vi "Reactor.vi"() -> ()   [LabVIEW 2017, in "HMILibrary.lvlib"]
uses:
  HMILibrary.lvlib
  <vilib>/Platform/TimedLoop/XDataNode/timing_clust.ctl
  <vilib>/Platform/TimedLoop/XDataNode/nitl_modes.ctl
  <vilib>/Platform/TimedLoop/XDataNode/wakeup.ctl
  <vilib>/Utility/file.llb/Write Delimited Spreadsheet (string).vi
  <vilib>/Utility/file.llb/Write Delimited Spreadsheet (DBL).vi
  <vilib>/platform/TimedLoop/XDataNode/XDataNode.xnode
  <vilib>/Platform/TimedLoop/XDataNode/XDNodeRunTimeDep.lvlib
panel:
  out "Hot Leg Temp":dbl
  out "color2":u32(colorbox)
  in  "Reactor\nPower":dbl(slide) scale=10.0..10000.0
  out "Heater Outlet Temp":dbl caption="C"
  out "Primary HX Outlet Temp":dbl
  out "Cold Leg Temp":dbl
  in  "stop":bool
  out "Warnings":string
  out "color1":u32(colorbox)
  in  "Tthreshold1":dbl=0.588
  in  "Tthreshold2":dbl=0.5934
  in  "Tthreshold3":dbl=1.6494
  in  "Tthreshold4":dbl=0.4812
  in  "dTthreshold1":dbl=2.361
  in  "dTthreshold2":dbl=2.6736
  in  "dTthreshold3":dbl=2.8362
  in  "dTthreshold4":dbl=2.1702
  in  "Tsamplethreshold":dbl=3.0
  in  "dTsamplethreshold":dbl=10.0
  out "color3":u32(colorbox)
  out "color4":u32(colorbox)
  out "Sensor 1":cluster{"placeholder1":dbl, dbl}(graph)
  out "Sensor 2":cluster{"placeholder1":dbl, dbl}(graph)
  out "Sensor 3":cluster{"placeholder1":dbl, dbl}(graph)
  out "Sensor 4":cluster{"placeholder1":dbl, dbl}(graph)
  in  "Hold Model Inputs Constant":bool
  in  "Clear Warnings":bool
  in  "Weight of measured values in filter":dbl=0.01
  # "Reactor and Primary Loop"
  # "Primary Heat\nExchanger"
  # "Reactor"
  # "Pump"
  # "Temperatures in degrees C"
  # "Fault Detection"
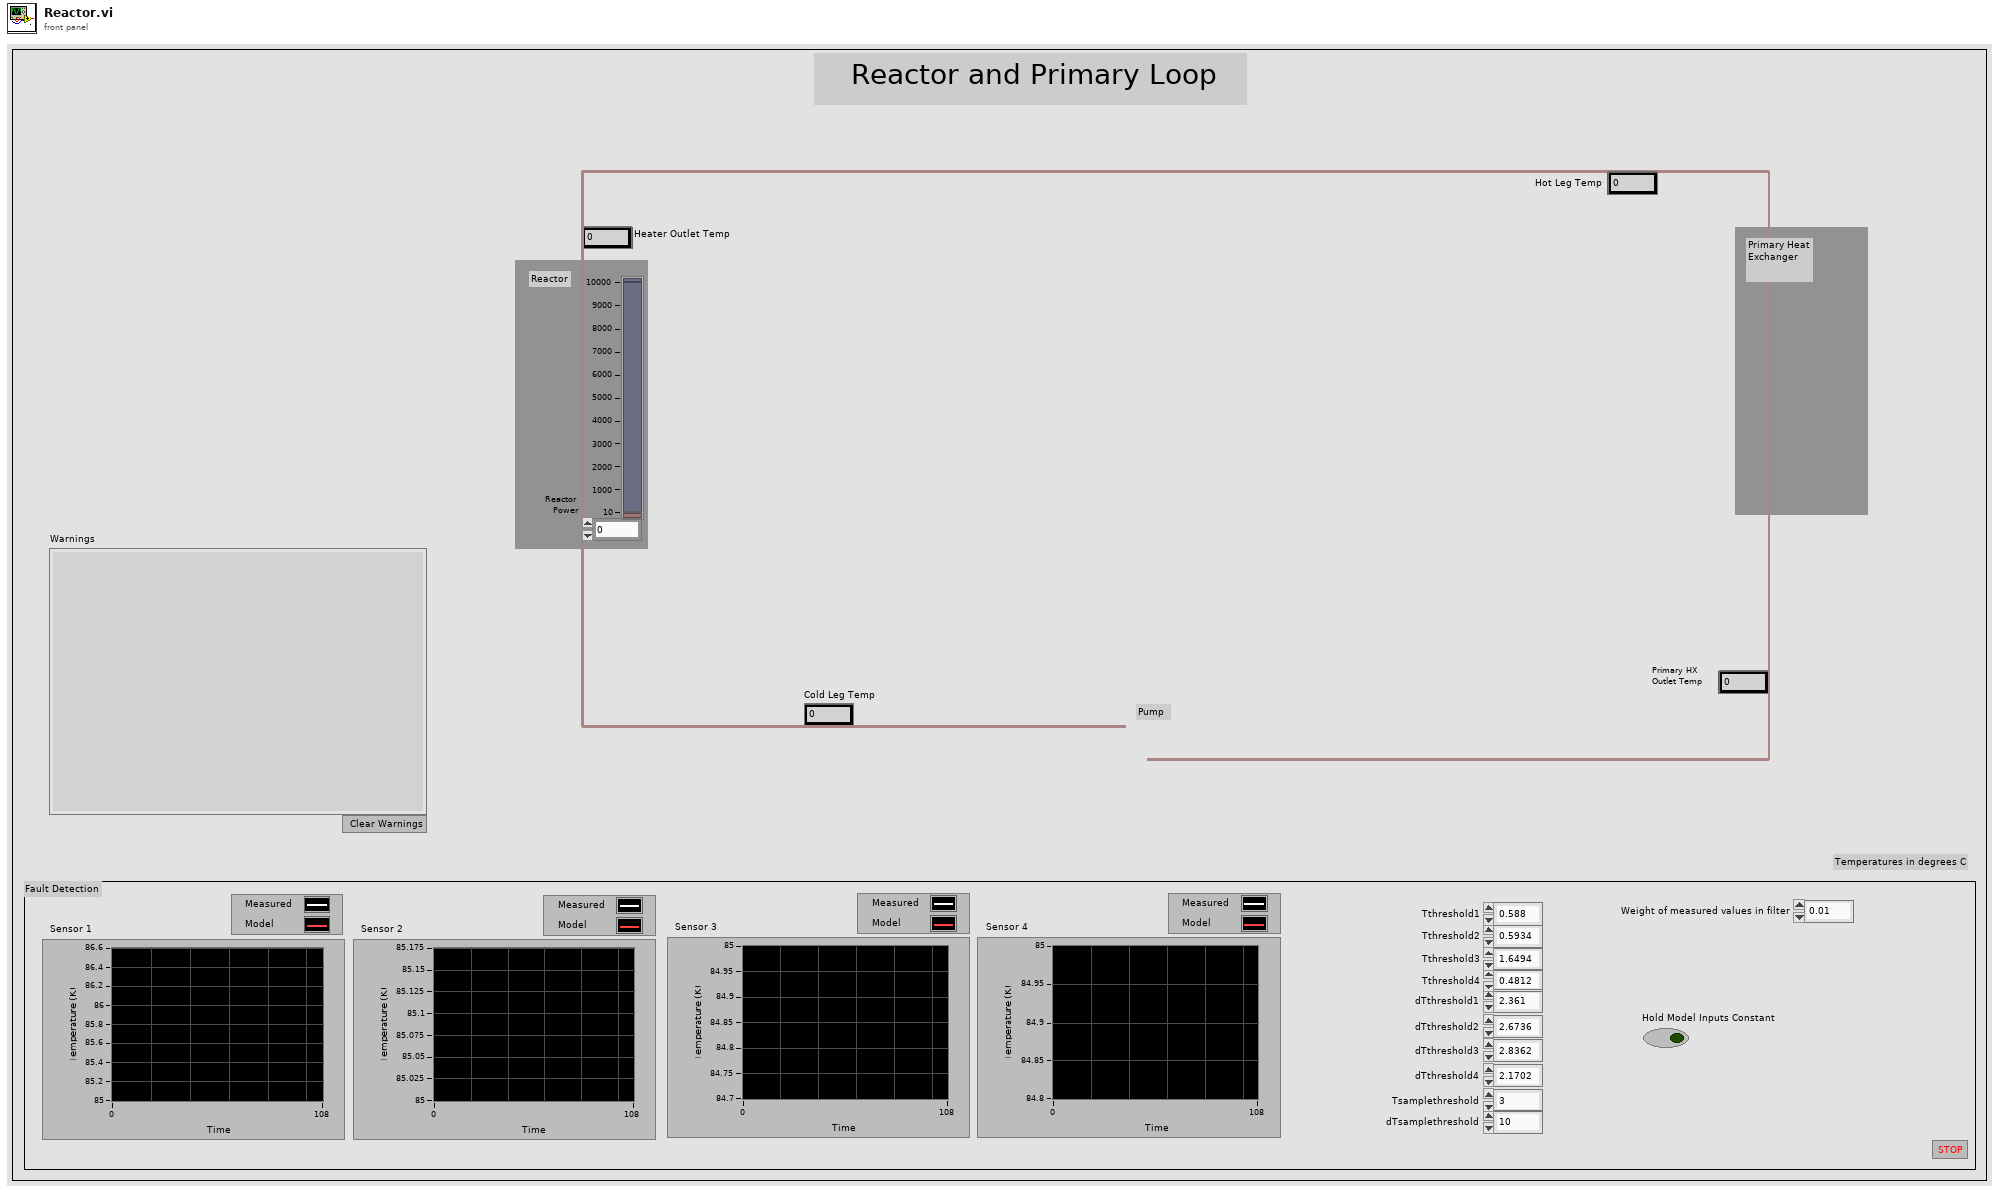
[diagram p1: front panel]
types:
  T1 = typedef "XDNodeRunTimeDep.lvlib/timing_clust.ctl" = cluster{"Expected End [f-1]":u64, "Actual End [f-1]":u64, "Finished Late? [f-1]":bool, "Expected End [i-1]":u64, "Actual End [i-1]":u64, "Finished Late? [i-1]":bool, "Expected Start [i]":u64, "Actual Start [i]":u64, "Expected Start [f]":u64, "Actual Start [f]":u64, "Source Name":string, "Structure Name":string, "Period":i64, "Deadline":i64, "Offset":i64, "Start":i64, "Priority":i32, "Timeout":i32, "Mode":T2, "Wakeup Reason":T3, "Error":errorcluster, "Source Type":string, "Secondary Source Type":string, "Global End Time":u64, "Global Start Time":u64, "Frame Duration":u64, "Iteration Duration":u64, "Assigned CPU":i32, "I/O Scan Engine Mode":u32}
  T2 = typedef "XDNodeRunTimeDep.lvlib/nitl_modes.ctl" = enum32{"No Change", "Process missed periods, maintain original phase", "Discard missed periods, maintain original phase", "Process missed periods, ignore original phase", "Discard missed periods, ignore original phase"}
  T3 = typedef "XDNodeRunTimeDep.lvlib/wakeup.ctl" = enum32{"Normal", "Aborted", "Asynchronous wakeup", "Timing source error", "Timed loop error", "Timeout"}
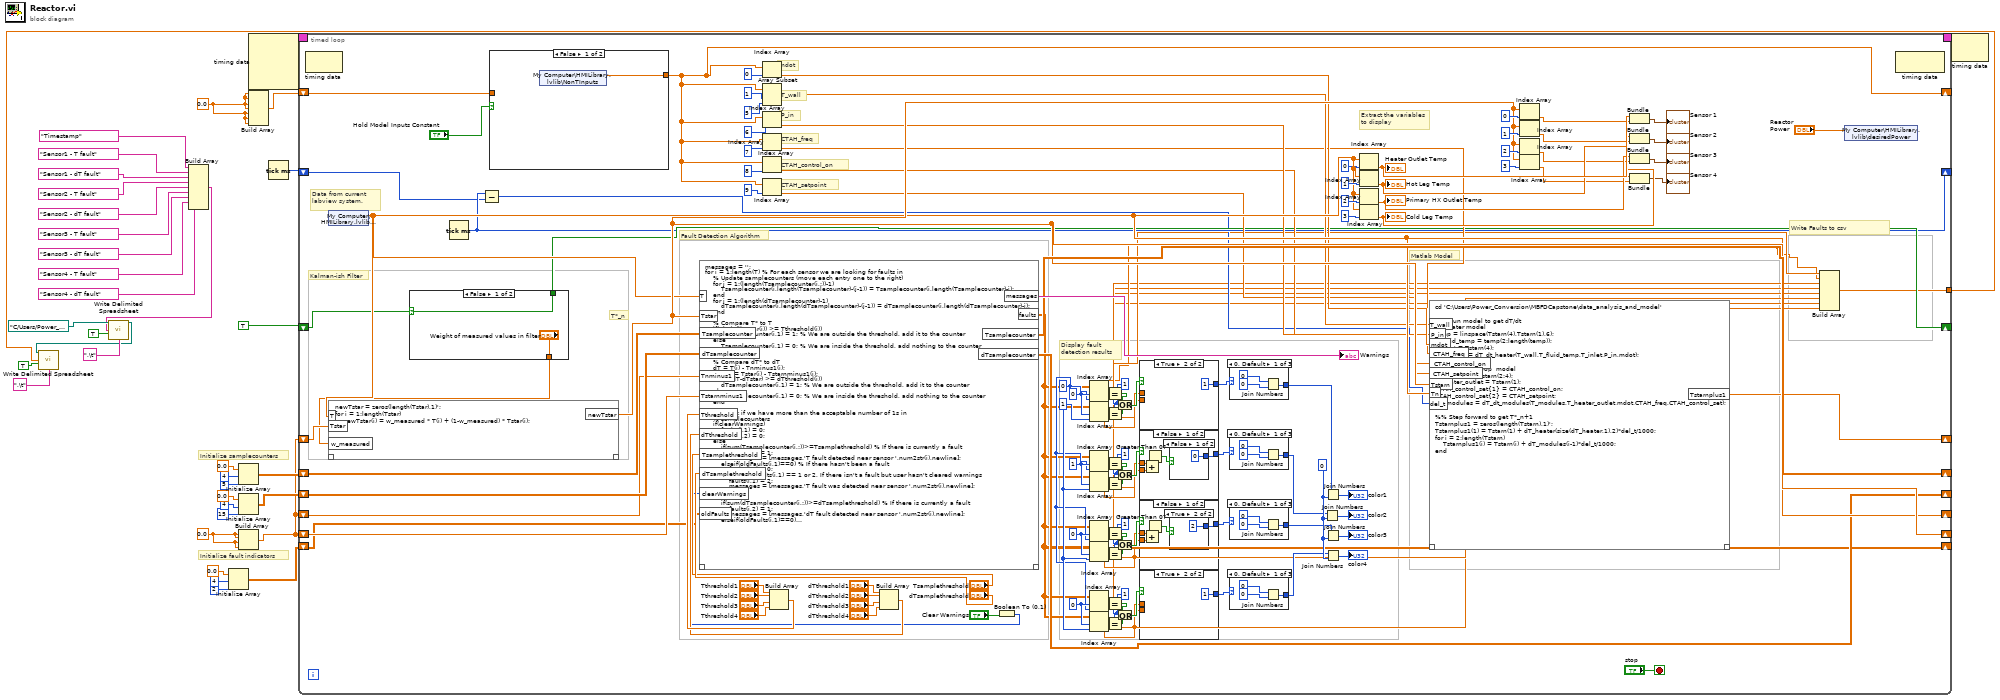
[diagram p0: block diagram]
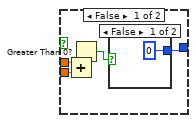
[diagram p2: hidden frame]
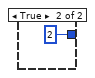
[diagram p3: hidden frame]
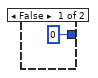
[diagram p4: hidden frame]
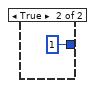
[diagram p5: hidden frame]
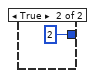
[diagram p6: hidden frame]
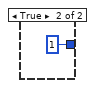
[diagram p7: hidden frame]
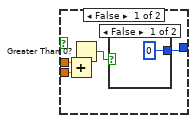
[diagram p8: hidden frame]
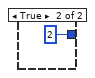
[diagram p9: hidden frame]
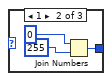
[diagram p10: hidden frame]
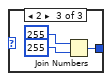
[diagram p11: hidden frame]
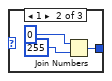
[diagram p12: hidden frame]
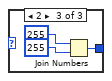
[diagram p13: hidden frame]
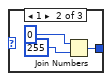
[diagram p14: hidden frame]
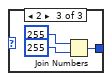
[diagram p15: hidden frame]
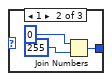
[diagram p16: hidden frame]
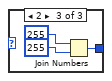
[diagram p17: hidden frame]
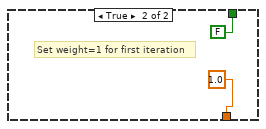
[diagram p18: hidden frame]
diagram:
  w24 = 0.0
  w27 = 0.0
  # "Initialize fault indicators"
  # "Initialize samplecounters"
  n1 = Build Array("Timestamp", "Sensor1 - T fault", "Sensor1 - dT fault", "Sensor2 - T fault", "Sensor2 - dT fault", "Sensor3 - T fault", "Sensor3 - dT fault", "Sensor4 - T fault", "Sensor4 - dT fault") -> (w1:string[])
  n2 = call-poly <vilib>:"Write Delimited Spreadsheet.vi"("file path (dialog if empty)"=path "C:/Users/Power_Conversion/Desktop", "1D data"=w1, "append to file? (new file:F)"=TRUE, "delimiter (\\t)"=",\t" ("delimiter (\\t)")) -> ("new file path (Not A Path if cancelled)"=w13:path)  [unwired: 10 in, 1 out]
  n3 = Initialize Array(0.0, 4, 2) -> (w21:dbl[][])
  n4 = Initialize Array(0.0, 4, 5) -> (w33:dbl[][])
  n5 = Initialize Array(0.0, 4, 15) -> (w32:dbl[][])
  n6 = Build Array(w27, w27, w27, w27) -> (w26:dbl[])
  n7 = node-c288() -> (w37:T1)  [unwired: 4 in]
  n8 = Build Array(w24, w24, w24, w24, w24, w24, w24) -> (w25:dbl[])
  n9 = Tick Count (ms)() -> (millisecond timer value=w18:u32)
  n10 = timed-loop {
    shift-right: [w140] -> _
    shift-left: w26 -> [w139]
    shift-right: [w145] -> _
    shift-left: w33 -> [w144]
    shift-right: [w53] -> _
    shift-left: w32 -> [w143]
    shift-right: [w105] -> _
    shift-left: w26 -> [w142]
    shift-right: [w118] -> _
    shift-left: w26 -> [w141]
    timing: w37 -> [_]
    timing-out: [_] -> w36
    shift-right: [w86] -> _
    shift-left: w25 -> [w90]
    shift-right: [w47] -> _
    shift-left: w21 -> [w87]
    shift-right: [w84] -> _
    shift-left: TRUE -> [w85]
    shift-right: [w82] -> _
    shift-left: w18 -> [w81]
    tunnel: [w39] -> w17
    stop <- "stop" stop-if-true
    w57 = 1
    w58 = 0
    w62 = 1
    w63 = 0
    w68 = 1
    w69 = 1
    w73 = 1
    w52 = 1
    w123 = u8 0
    w51 = 0
    w75 = 0
    # "Write Faults to csv"
    # "CTAH_setpoint"
    # "CTAH_control_on"
    # "CTAH_freq"
    # "P_in"
    # "T_wall"
    # "mdot"
    # "Kalman-ish Filter"
    # "Extract the variables to display"
    # "Data from current labview system."
    # "Display fault detection results"
    # "Fault Detection Algorithm"
    # "T*_n"
    # "Matlab Model"
    n11 = node-c288() -> ()  [unwired: 1 in, 1 out]
    n12 = shared-variable "My Computer\\HMILibrary.lvlib\\T_n"() -> (w105:dbl[])  [unwired: 1 in, 1 out]
    n13 = case shown="False" w85 {
      selector: w85 -> [w222 _]
      tunnel: [w222 FALSE] -> w84
      tunnel: ["Weight of measured values in filter" 1.0] -> w83
      frame False {
      }
      frame True {
        # "Set weight=1 for first iteration"
      }
    }
    n14 = script code="newTstar = zeros(length(Tstar),1)';\nfor i = 1:length(Tstar)\n    newTstar(i) = w_measured * T(i) + (1-w_measured) * Tstar(i);\nend"("T"=w105, "Tstar"=w139, "w_measured"=w83) -> ("newTstar"=w118:dbl[])  [unwired: 1 in, 1 out]
    n15 = Tick Count (ms)() -> (millisecond timer value=w82:u32)
    n16 = Subtract(x=w82, y=w81) -> (x-y=w80:u32)
    n17 = case shown="False" "Hold Model Inputs Constant" {
      tunnel: [w225 w226] -> w86
      tunnel: w90 -> [_ w226]
      frame False {
        n18 = shared-variable "My Computer\\HMILibrary.lvlib\\NonTInputs"() -> (w225:dbl[])  [unwired: 1 in, 1 out]
      }
      frame True {
      }
    }
    n19 = Index Array(array=w86, index=0) -> (element=w104:dbl)
    n20 = Array Subset(array=w86, index=1, length=5) -> (w100:dbl[])
    n21 = Index Array(array=w86, index=6) -> (element=w99:dbl)
    n22 = Index Array(array=w86, index=7) -> (element=w96:dbl)
    n23 = Index Array(array=w86, index=8) -> (element=w95:dbl)
    n24 = Index Array(array=w86, index=9) -> (element=w93:dbl)
    n25 = Build Array("Tthreshold1", "Tthreshold2", "Tthreshold3", "Tthreshold4") -> (w134:dbl[])
    n26 = Build Array("dTthreshold1", "dTthreshold2", "dTthreshold3", "dTthreshold4") -> (w129:dbl[])
    n27 = Boolean To (0,1)(Boolean="Clear Warnings") -> (0, 1=w88:i16)
    n28 = script code="messages = '';\nfor i = 1:length(T) % For each sensor we are looking for faults in\n    % Update samplecounters (move each entry one to the right)\n    for j = 1:(length(Tsamplecounter(i,:))-1)\n        Tsamplecounter(i,length(Tsamplecounter)-(j-1)) = Tsamplecounter(i,length(Tsamplecounter)-j);\n    end\n    for j = 1:(length(dTsamplecounter)-1)\n        dTsamplecounter(i,length(dTsamplecounter)-(j-1)) = dTsamplecounter(i,length(dTsamplecounter)-j);\n    end\n    \n    % Compare T* to T\n    if(abs(T(i)-Tstar(i)) >= Tthreshold(i))\n        Tsamplecounter(i,1) = 1; % We are outside the threshold, add it to the counter\n    else\n        Tsamplecounter(i,1) = 0; % We are inside the threshold, add nothing to the counter\n    end\n    \n    % Compare dT* to dT\n    dT = T(i) - Tnminus1(i);\n    dTstar = Tstar(i) - Tstarnminus1(i);\n    if(abs(dT-dTstar) >= dTthreshold(i))\n        dTsamplecounter(i,1) = 1; % We are outside the threshold, add it to the counter\n    else\n        dTsamplecounter(i,1) = 0; % We are inside the threshold, add nothing to the counter\n    end\n    \n    % Check if we have more than the acceptable number of 1s in\n    % samplecounters\n    if(clearWarnings)\n        faults(i,1) = 0;\n        faults(i,2) = 0;\n    else\n        if(sum(Tsamplecounter(i,:))>=Tsamplethreshold) % If there is currently a fault\n            faults(i,1) = 1;\n            messages = [messages,'T fault detected near sensor ',num2str(i),newline];\n        elseif(oldFaults(i,1)==0) % If there hasn't been a fault\n            faults(i,1) = 0;\n        else % oldFaults(i,1) == 1 or 2, If there isn't a fault but user hasn't cleared warnings\n            faults(i,1) = 2;\n            messages = [messages,'T fault was detected near sensor ',num2str(i),newline];\n        end\n        \n        if(sum(dTsamplecounter(i,:))>=dTsamplethreshold) % If there is currently a fault\n            faults(i,2) = 1;\n            messages = [messages,'dT fault detected near sensor ',num2str(i),newline];\n        elseif(oldFaults(i,1)==0) % If there hasn't been a fault\n            faults(i,2) = 0;\n        else % oldFaults(i,1) == 1 or 2, If there isn't a fault but user hasn't cleared warnings\n            faults(i,2) = 2;\n            messages = [messages,'dT fault was detected near sensor ',num2str(i),newline];\n        end\n    end\nend"("T"=w105, "Tstar"=w118, "Tsamplecounter"=w144, "dTsamplecounter"=w143, "Tnminus1"=w142, "Tstarnminus1"=w141, "Tthreshold"=w134, "dTthreshold"=w129, "Tsamplethreshold"="Tsamplethreshold", "dTsamplethreshold"="dTsamplethreshold", "clearWarnings"=w88, "oldFaults"=w87) -> ("faults"=w47:dbl[][], "messages"=→"Warnings":string, "Tsamplecounter"=w145:dbl[][], "dTsamplecounter"=w53:dbl[][])  [unwired: 1 in, 1 out]
    n29 = Index Array(array=w47, index (row)=w75, index (col)=w51) -> (element=w48:dbl)
    n30 = Index Array(array=w47, index (row)=w75, index (col)=w52) -> (element=w46:dbl)
    n31 = Index Array(array=w47, index (row)=w69, index (col)=w51) -> (element=w45:dbl)
    n32 = Index Array(array=w47, index (row)=w69, index (col)=w52) -> (element=w44:dbl)
    n33 = Index Array(array=w47, index (row)=w63, index (col)=w51) -> (element=w43:dbl)
    n34 = Index Array(array=w47, index (row)=w63, index (col)=w52) -> (element=w42:dbl)
    n35 = Index Array(array=w47, index (row)=w58, index (col)=w51) -> (element=w41:dbl)
    n36 = Index Array(array=w47, index (row)=w58, index (col)=w52) -> (element=w40:dbl)
    n37 = Equal?(x=w73, y=w48) -> (x = y?=w71:bool)
    n38 = Equal?(x=w73, y=w46) -> (x = y?=w72:bool)
    n39 = Equal?(x=w68, y=w45) -> (x = y?=w66:bool)
    n40 = Equal?(x=w68, y=w44) -> (x = y?=w67:bool)
    n41 = Equal?(x=w62, y=w43) -> (x = y?=w60:bool)
    n42 = Equal?(x=w62, y=w42) -> (x = y?=w61:bool)
    n43 = Equal?(x=w57, y=w41) -> (x = y?=w55:bool)
    n44 = Equal?(x=w57, y=w40) -> (x = y?=w56:bool)
    n45 = Or(x=w71, y=w72) -> (x .or. y?=w70:bool)
    n46 = Or(x=w66, y=w67) -> (x .or. y?=w65:bool)
    n47 = Or(x=w60, y=w61) -> (x .or. y?=w59:bool)
    n48 = Or(x=w55, y=w56) -> (x .or. y?=w54:bool)
    n49 = case shown="True" w70 {
      tunnel: [w177 1] -> w74
      tunnel: w48 -> [w181 _]
      tunnel: w46 -> [w180 _]
      frame False {
        n50 = Add(x=w181, y=w180) -> (x+y=w178:dbl)
        n51 = Greater Than 0?(x=w178) -> (x > 0?=w179:bool)
        n52 = case shown="False" w179 {
          tunnel: [0 2] -> w177
          frame False {
          }
          frame True {
          }
        }
      }
      frame True {
      }
    }
    n53 = case shown="False" w65 {
      tunnel: [w169 1] -> w64
      tunnel: w45 -> [w173 _]
      tunnel: w44 -> [w172 _]
      frame False {
        n54 = Add(x=w173, y=w172) -> (x+y=w170:dbl)
        n55 = Greater Than 0?(x=w170) -> (x > 0?=w171:bool)
        n56 = case shown="False" w171 {
          tunnel: [0 2] -> w169
          frame False {
          }
          frame True {
          }
        }
      }
      frame True {
      }
    }
    n57 = case shown="False" w59 {
      tunnel: [w161 1] -> w49
      tunnel: w43 -> [w165 _]
      tunnel: w42 -> [w164 _]
      frame False {
        n58 = Add(x=w165, y=w164) -> (x+y=w162:dbl)
        n59 = Greater Than 0?(x=w162) -> (x > 0?=w163:bool)
        n60 = case shown="True" w163 {
          tunnel: [0 2] -> w161
          frame False {
          }
          frame True {
          }
        }
      }
      frame True {
      }
    }
    n61 = case shown="True" w54 {
      tunnel: [w153 1] -> w50
      tunnel: w41 -> [w157 _]
      tunnel: w40 -> [w156 _]
      frame False {
        n62 = Add(x=w157, y=w156) -> (x+y=w154:dbl)
        n63 = Greater Than 0?(x=w154) -> (x > 0?=w155:bool)
        n64 = case shown="False" w155 {
          tunnel: [0 2] -> w153
          frame False {
          }
          frame True {
          }
        }
      }
      frame True {
      }
    }
    n65 = case shown="0, Default" w74 {
      tunnel: [w212 w215 w218] -> w79
      frame 0, Default {
        n66 = Join Numbers(hi=u8 0, lo=u8 0) -> ((hi.lo)=w212:u16)
      }
      frame 1 {
        n67 = Join Numbers(hi=u8 0, lo=u8 255) -> ((hi.lo)=w215:u16)
      }
      frame 2 {
        n68 = Join Numbers(hi=u8 255, lo=u8 255) -> ((hi.lo)=w218:u16)
      }
    }
    n69 = case shown="0, Default" w64 {
      tunnel: [w203 w206 w209] -> w78
      frame 0, Default {
        n70 = Join Numbers(hi=u8 0, lo=u8 0) -> ((hi.lo)=w203:u16)
      }
      frame 1 {
        n71 = Join Numbers(hi=u8 0, lo=u8 255) -> ((hi.lo)=w206:u16)
      }
      frame 2 {
        n72 = Join Numbers(hi=u8 255, lo=u8 255) -> ((hi.lo)=w209:u16)
      }
    }
    n73 = case shown="0, Default" w49 {
      tunnel: [w194 w197 w200] -> w77
      frame 0, Default {
        n74 = Join Numbers(hi=u8 0, lo=u8 0) -> ((hi.lo)=w194:u16)
      }
      frame 1 {
        n75 = Join Numbers(hi=u8 0, lo=u8 255) -> ((hi.lo)=w197:u16)
      }
      frame 2 {
        n76 = Join Numbers(hi=u8 255, lo=u8 255) -> ((hi.lo)=w200:u16)
      }
    }
    n77 = case shown="0, Default" w50 {
      tunnel: [w185 w188 w191] -> w76
      frame 0, Default {
        n78 = Join Numbers(hi=u8 0, lo=u8 0) -> ((hi.lo)=w185:u16)
      }
      frame 1 {
        n79 = Join Numbers(hi=u8 0, lo=u8 255) -> ((hi.lo)=w188:u16)
      }
      frame 2 {
        n80 = Join Numbers(hi=u8 255, lo=u8 255) -> ((hi.lo)=w191:u16)
      }
    }
    n81 = Join Numbers(hi=w78, lo=w123) -> ((hi.lo)=→"color2":u32)
    n82 = Join Numbers(hi=w79, lo=w123) -> ((hi.lo)=→"color1":u32)
    n83 = Join Numbers(hi=w77, lo=w123) -> ((hi.lo)=→"color3":u32)
    n84 = Join Numbers(hi=w76, lo=w123) -> ((hi.lo)=→"color4":u32)
    n85 = Index Array(array=w105, index=0) -> (element=w117:dbl)
    "Heater Outlet Temp" <- w117
    n86 = Index Array(array=w105, index=1) -> (element=w116:dbl)
    "Hot Leg Temp" <- w116
    n87 = Index Array(array=w105, index=2) -> (element=w115:dbl)
    "Primary HX Outlet Temp" <- w115
    n88 = Index Array(array=w105, index=3) -> (element=w114:dbl)
    "Cold Leg Temp" <- w114
    n89 = script code="cd 'C:\\Users\\Power_Conversion\\MBFDCapstone\\data_analysis_and_model'\n\n%% Run model to get dT/dt\n% Heater model\ntemp = linspace(Tstarn(4),Tstarn(1),6);\nT_fluid_temp = temp(2:length(temp));\nT_inlet = Tstarn(4);\ndT_heater = dT_dt_heater(T_wall,T_fluid_temp,T_inlet,P_in,mdot);\n\n% Rest of the loop  model\nT_modules = Tstarn(2:4);\nT_heater_outlet = Tstarn(1);\nCTAH_control_set{1} = CTAH_control_on;\nCTAH_control_set{2} = CTAH_setpoint;\ndT_modules = dT_dt_modules(T_modules,T_heater_outlet,mdot,CTAH_freq,CTAH_control_set);\n\n%% Step forward to get T*_n+1\nTstarnplus1 = zeros(length(Tstarn),1)';\nTstarnplus1(1) = Tstarn(1) + dT_heater(size(dT_heater,1),2)*del_t/1000;\nfor i = 2:length(Tstarn)\n    Tstarnplus1(i) = Tstarn(i) + dT_modules(i-1)*del_t/1000;\nend"("Tstarn"=w118, "T_wall"=w100, "P_in"=w99, "mdot"=w104, "Tn"=w105, "CTAH_freq"=w96, "CTAH_control_on"=w95, "CTAH_setpoint"=w93, "del_t"=w80) -> ("Tstarnplus1"=w140:dbl[])  [unwired: 1 in, 1 out]
    n90 = Index Array(array=w118, index=0) -> (element=w113:dbl)
    n91 = Index Array(array=w118, index=1) -> (element=w112:dbl)
    n92 = Index Array(array=w118, index=2) -> (element=w111:dbl)
    n93 = Index Array(array=w118, index=3) -> (element=w110:dbl)
    n94 = Bundle("Numeric"=w117, w113) -> (→"Sensor 1":cluster{"Numeric":dbl, dbl})  [unwired: 1 in]
    n95 = Bundle("Numeric"=w116, w112) -> (→"Sensor 2":cluster{"Numeric":dbl, dbl})  [unwired: 1 in]
    n96 = Bundle("Numeric"=w115, w111) -> (→"Sensor 3":cluster{"Numeric":dbl, dbl})  [unwired: 1 in]
    n97 = Bundle("Numeric"=w114, w110) -> (→"Sensor 4":cluster{"Numeric":dbl, dbl})  [unwired: 1 in]
    n98 = Build Array(w48, w46, w45, w44, w43, w42, w41, w40) -> (w39:dbl[])
    n99 = shared-variable "My Computer\\HMILibrary.lvlib\\desiredPower"("Reactor\nPower") -> ()  [unwired: 1 in, 1 out]
    n100 = node-c288() -> ()  [unwired: 1 in, 1 out]
  }
  n101 = call-poly <vilib>:"Write Delimited Spreadsheet.vi"("file path (dialog if empty)"=w13, "1D data"=w17, "append to file? (new file:F)"=TRUE, "delimiter (\\t)"=",\t" ("delimiter (\\t)")) -> ()  [unwired: 10 in, 2 out]
  n102 = node-c288(w36) -> ()  [unwired: 1 out]
